vi "rethinkdb_example_test2.vi"() -> ()   [LabVIEW 2017]
uses:
  rethinkdb/reql_db_create.vi
  rethinkdb/reql_db_list.vi
  rethinkdb/reql_table_create.vi
  rethinkdb/reql_table_list.vi
  rethinkdb/reql_item_insert.vi
  rethinkdb/reql_item_get.vi
  rethinkdb/reql_table_drop.vi
  rethinkdb/reql_db_drop.vi
  rethinkdb/RethinkDB.lvclass
  rethinkdb/rethinkdb.lvlib
panel:
  out "state":T1(ring)
  in  "ms throttle":u32=1000
  out "db exists?":bool
  out "table exists?":bool
  in  "table name":string="MyTable"
  in  "db name":string="MyDB"
  in  "actions":T2={"0:db_create"=TRUE, "1:table_create"=TRUE, "2:insert"=TRUE, "3:table_drop"=FALSE, "4:db_drop"=FALSE}
  out "value":variant
  in  "insert":T3={"mybool"=TRUE, "myint"=-123, "myuint"=4567, "myfloat"=3.1415, "mystring"="hello\nworld", "my\nArray"=[1, 2, 3], "obj\"array"=[{"b"=TRUE}, {"b"=FALSE}], "subcluster"={"float_nan"=nan, "i8"=-128, "float+inf"=inf, "float-inf"=-inf}}
  out "debug":string
  out "table list":string[](array[string])
  out "db list":string[](array[string])
  out "error out":errorcluster
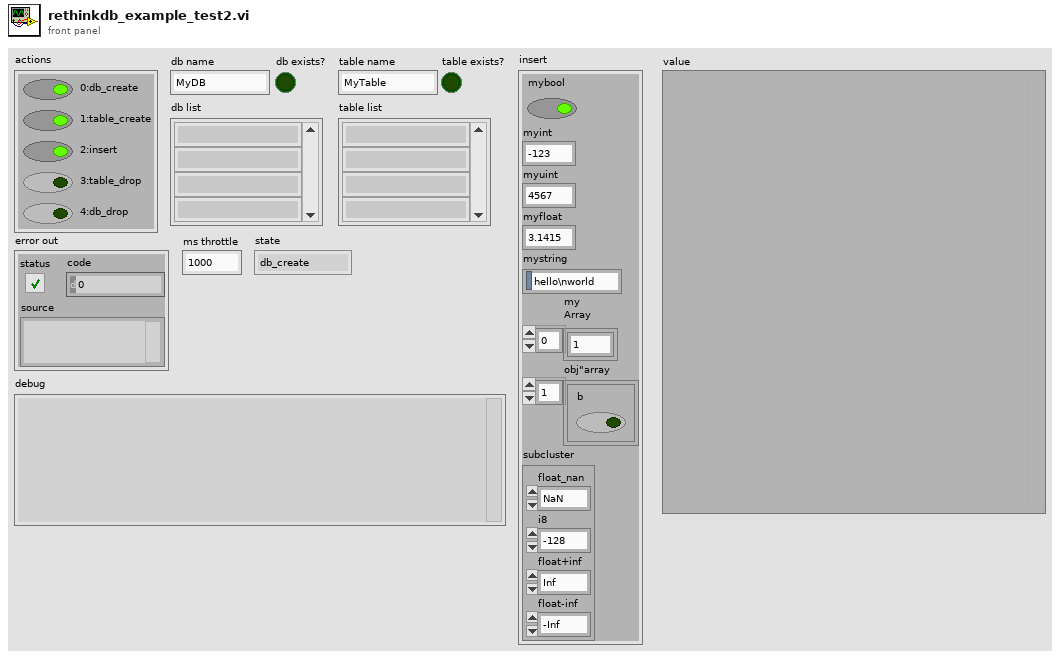
[diagram p1: front panel]
types:
  T1 = enum8{"db_create", "table_create", "insert", "table_drop", "db_drop", "done"}
  T2 = cluster{"0:db_create":bool, "1:table_create":bool, "2:insert":bool, "3:table_drop":bool, "4:db_drop":bool}
  T3 = cluster{"mybool":bool, "myint":i32, "myuint":u16, "myfloat":dbl, "mystring":string, "my\nArray":u8[], "obj\"array":cluster{"b":bool}[], "subcluster":cluster{"float_nan":dbl, "i8":i8, "float+inf":dbl, "float-inf":dbl}}
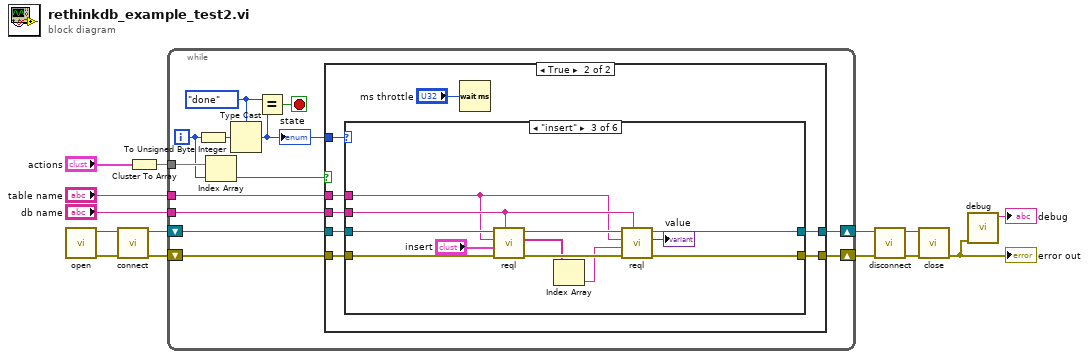
[diagram p0: block diagram]
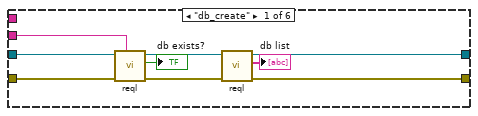
[diagram p3: hidden frame]
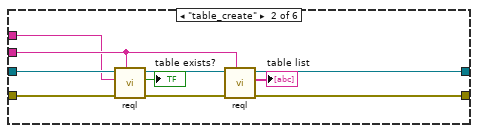
[diagram p4: hidden frame]
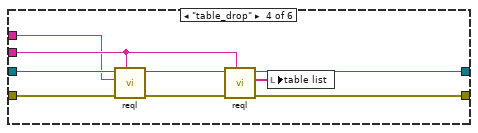
[diagram p5: hidden frame]
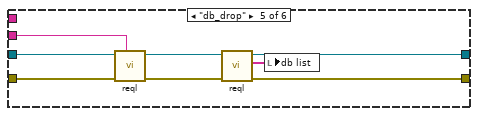
[diagram p6: hidden frame]
diagram:
  n1 = call "open.vi"() -> ("error out"=w14:errorcluster, "rethinkdb out"=w13:refnum<class "RethinkDB.lvclass">)  [unwired: 10 in]
  n2 = call "connect.vi"("error in (no error)"=w14, "rethinkdb in"=w13) -> ("error out"=w8:errorcluster, "rethinkdb out"=w7:refnum<class "RethinkDB.lvclass">)  [unwired: 8 in]
  n3 = Cluster To Array(cluster="actions") -> (array=w5:bool[])
  n4 = while {
    tunnel: w5 -> [w27]
    tunnel: "db name" -> [w22]
    tunnel: "table name" -> [w21]
    shift-right: [w23] -> w2
    shift-left: w7 -> [w26]
    shift-right: [w24] -> w1
    shift-left: w8 -> [w25]
    i -> [w18]
    stop <- w15 stop-if-true
    w16 = T1."done" ("x")
    n5 = To Unsigned Byte Integer(number=w18) -> (unsigned 8bit integer=w20:u8)
    n6 = Index Array(array=w27, index=w18) -> (element=w19:bool)
    n7 = Type Cast(type=w16, x=w20) -> (*(type *) &x=w17:T1)
    "state" <- w17
    n8 = Equal?(x=w16, y=w17) -> (x = y?=w15:bool)
    n9 = case shown="True" w19 {
      tunnel: w17 -> [_ w37]
      tunnel: w26 -> [w28 w36]
      tunnel: w25 -> [w29 w35]
      tunnel: [w29 w34] -> w24
      tunnel: [w28 w33] -> w23
      tunnel: w22 -> [_ w32]
      tunnel: w21 -> [_ w31]
      frame False {
      }
      frame True {
        n10 = case shown="\"insert\"" w37 {
          tunnel: w36 -> [w42 w52 w65 w74 w82 w87]
          tunnel: w35 -> [w43 w53 w66 w75 w83 w86]
          tunnel: [w41 w50 w63 w72 w81 w86] -> w34
          tunnel: [w40 w51 w64 w73 w80 w87] -> w33
          tunnel: w32 -> [w39 w49 w62 w71 w79 _]
          tunnel: w31 -> [_ w48 w59 w70 _ _]
          frame "db_create" {
            n11 = call-poly "reql.vi"("db name"=w39, "error in (no error)"=w43, "rethinkdb in"=w42) -> ("error out"=w45:errorcluster, "db exists?"=→"db exists?":bool, "rethinkdb out"=w44:refnum<class "RethinkDB.lvclass">)  [unwired: 5 in, 1 out]
            n12 = call-poly "reql.vi"("error in (no error)"=w45, "rethinkdb in"=w44) -> ("error out"=w41:errorcluster, "db list"=→"db list":string[], "rethinkdb out"=w40:refnum<class "RethinkDB.lvclass">)  [unwired: 6 in, 1 out]
          }
          frame "table_create" {
            n13 = call-poly "reql.vi"("db name"=w49, "error in (no error)"=w53, "table name"=w48, "rethinkdb in"=w52) -> ("error out"=w54:errorcluster, "table exists?"=→"table exists?":bool, "rethinkdb out"=w55:refnum<class "RethinkDB.lvclass">)  [unwired: 4 in, 1 out]
            n14 = call-poly "reql.vi"("db name"=w49, "error in (no error)"=w54, "rethinkdb in"=w55) -> ("error out"=w50:errorcluster, "table list"=→"table list":string[], "rethinkdb out"=w51:refnum<class "RethinkDB.lvclass">)  [unwired: 5 in, 1 out]
          }
          frame "insert" {
            n15 = call-poly "reql.vi"("db name"=w62, "error in (no error)"=w66, "object"="insert", "table name"=w59, "rethinkdb in"=w65) -> ("error out"=w67:errorcluster, "generated keys"=w61:string[], "rethinkdb out"=w68:refnum<class "RethinkDB.lvclass">)  [unwired: 3 in, 1 out]
            n16 = Index Array(array=w61) -> (element=w60:string)  [unwired: 1 in]
            n17 = call-poly "reql.vi"("db name"=w62, "error in (no error)"=w67, "id"=w60, "table name"=w59, "rethinkdb in"=w68) -> ("error out"=w63:errorcluster, "value"=→"value":variant, "rethinkdb out"=w64:refnum<class "RethinkDB.lvclass">)  [unwired: 3 in, 1 out]
          }
          frame "table_drop" {
            n18 = call-poly "reql.vi"("db name"=w71, "error in (no error)"=w75, "table name"=w70, "rethinkdb in"=w74) -> ("error out"=w76:errorcluster, "rethinkdb out"=w77:refnum<class "RethinkDB.lvclass">)  [unwired: 4 in, 2 out]
            n19 = call-poly "reql.vi"("db name"=w71, "error in (no error)"=w76, "rethinkdb in"=w77) -> ("error out"=w72:errorcluster, "table list"=w69:string[], "rethinkdb out"=w73:refnum<class "RethinkDB.lvclass">)  [unwired: 5 in, 1 out]
            n20 = local write "table list"(w69) -> ()
          }
          frame "db_drop" {
            n21 = call-poly "reql.vi"("db name"=w79, "error in (no error)"=w83, "rethinkdb in"=w82) -> ("error out"=w85:errorcluster, "rethinkdb out"=w84:refnum<class "RethinkDB.lvclass">)  [unwired: 5 in, 2 out]
            n22 = call-poly "reql.vi"("error in (no error)"=w85, "rethinkdb in"=w84) -> ("error out"=w81:errorcluster, "db list"=w78:string[], "rethinkdb out"=w80:refnum<class "RethinkDB.lvclass">)  [unwired: 6 in, 1 out]
            n23 = local write "db list"(w78) -> ()
          }
          frame Default {
          }
        }
        n24 = Wait (ms)(milliseconds to wait="ms throttle") -> ()  [unwired: 1 out]
      }
    }
  }
  n25 = call "disconnect.vi"("error in (no error)"=w1, "rethinkdb in"=w2) -> ("error out"=w12:errorcluster, "rethinkdb out"=w11:refnum<class "RethinkDB.lvclass">)  [unwired: 8 in]
  n26 = call "close.vi"("error in (no error)"=w12, "rethinkdb in"=w11) -> ("error out"=w10:errorcluster)  [unwired: 9 in]
  "error out" <- w10
  n27 = call "debug.vi"("error in (no error)"=w10) -> ("debug"=→"debug":string)  [unwired: 9 in, 1 out]
